vi "ex_4.vi"() -> ()   [LabVIEW 2020]
panel:
  out "Numeric":i32
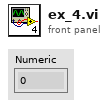
[diagram p1: front panel]
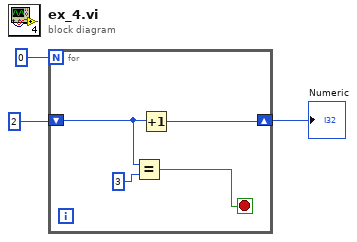
[diagram p0: block diagram]
diagram:
  n1 = for {
    N: 0 -> [_]
    shift-right: [w7] -> w1
    shift-left: 2 -> [w6]
    stop <- w4 stop-if-true
    n2 = Equal?(x=w6, y=3) -> (x = y?=w4:bool)
    n3 = Increment(x=w6) -> (x+1=w7:i32)
  }
  "Numeric" <- w1
